vi "verificarDatosVarilla.vi"(8 "error in":errorcluster, 11 "dataToWrite":T2) -> (0 "error out":errorcluster, 3 "dataToWriteModify":T1)   [LabVIEW 2014]
uses:
  <vilib>/addons/database/Auxilliary.llb/DB Tools Format Datetime String (Time Stamp).vi
  <vilib>/addons/database/NI_Database_API.lvlib
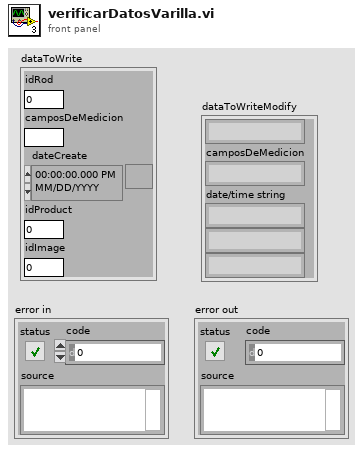
[diagram p1: front panel]
types:
  T1 = cluster{string, "camposDeMedicion":string, "date/time string":string, string, string}
  T2 = cluster{"idRod":dbl, "camposDeMedicion":string, "dateCreate":timestamp, "idProduct":dbl, "idImage":dbl}
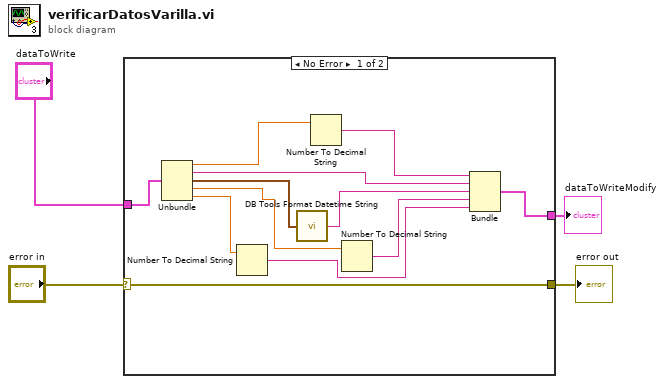
[diagram p0: block diagram]
diagram:
  n1 = case shown="No Error" "error in" {
    selector: "error in" -> [w11 w17]
    tunnel: "dataToWrite" -> [w16 _]
    tunnel: [w15 _] -> w1
    tunnel: [w11 w17] -> w3
    frame No Error {
      n2 = Unbundle(w16) -> ("idRod"=w13:dbl, "camposDeMedicion"=w12:string, "dateCreate"=w10:timestamp, "idProduct"=w8:dbl, "idImage"=w7:dbl)
      n3 = Number To Decimal String(number=w7) -> (decimal integer string=w5:string)  [unwired: 1 in]
      n4 = call-poly <vilib>:"DB Tools Format Datetime String.vi"("time stamp"=w10) -> ("date/time string"=w9:string)
      n5 = Number To Decimal String(number=w13) -> (decimal integer string=w14:string)  [unwired: 1 in]
      n6 = Number To Decimal String(number=w8) -> (decimal integer string=w6:string)  [unwired: 1 in]
      n7 = Bundle(w14, "camposDeMedicion"=w12, "date/time string"=w9, w6, w5) -> (w15:T1)  [unwired: 1 in]
    }
    frame Error {
    }
  }
  "error out" <- w3
  "dataToWriteModify" <- w1
